vi "EthernetIP_CompactLogix_Servo.vi"() -> ()   [LabVIEW 2013]
uses:
  <vilib>/ethernetip/ethernetip.lvlib
  <vilib>/ethernetip/ethernetip.llb/EthernetIP Tag Write BOOL.vi
  <vilib>/ethernetip/ethernetip.llb/EthernetIP Tag Write REAL.vi
  <vilib>/ethernetip/ethernetip.llb/EthernetIP Tag Write DINT.vi
  <vilib>/ethernetip/ethernetip.llb/EthernetIP Tag Read BOOL.vi
panel:
  in  "Number of Elements 2":u32=1
  out "Servo1 Fault":bool
  in  "Number of Elements":u32=1
  out "Servo1 Fault":bool[](array[boolean])
  out "Servo1 Enabled":bool
  in  "VelocityLimit(172.20.2.53)":dbl=100.0
  in  "DecelerationLimit(172.20.2.53)":dbl=500.0
  in  "AccelerationLimit(172.20.2.53)":dbl=500.0
  in  "VelocityLimit(172.20.2.52)":dbl=100.0
  in  "DecelerationLimit(172.20.2.52)":dbl=500.0
  in  "AccelerationLimit(172.20.2.52)":dbl=500.0
  in  "Reference Source(172.20.2.53)":u16(ring)=3 items=["current", "velocity", "incremental position", "absolute position", "incremental registration", "absolute registration"]
  in  "Reference Source(172.20.2.52)":u16(ring)=3 items=["current", "velocity", "incremental position", "absolute position", "incremental registration", "absolute registration"]
  out "난수 결과값":dbl
  in  "CommandPosition":dbl(slide) scale=0.0..7.5
  in  "Time Delay":i32(knob)=50 scale=0.0..1000.0
  in  "StartMotion SW":bool
  in  "정지 버튼":bool
  in  "Error In":errorcluster caption="에러 입력"
  out "Error Out":errorcluster caption="에러 출력"
  in  "타임아웃":i32(knob)=1000 scale=0.0..1000.0
  in  "Servo1 On SW":bool
  # "Servo1(172.20.2.53)"
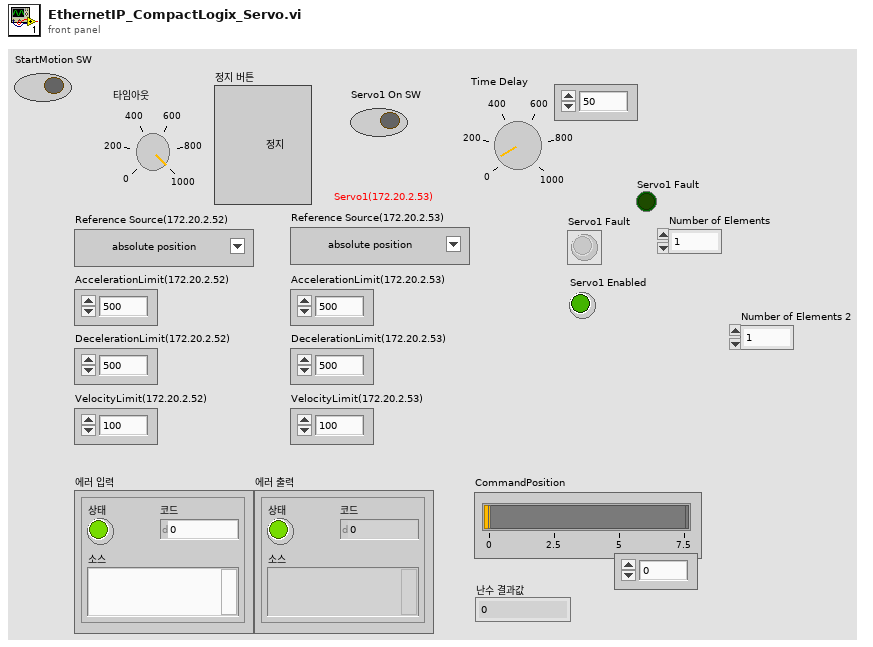
[diagram p1: front panel]
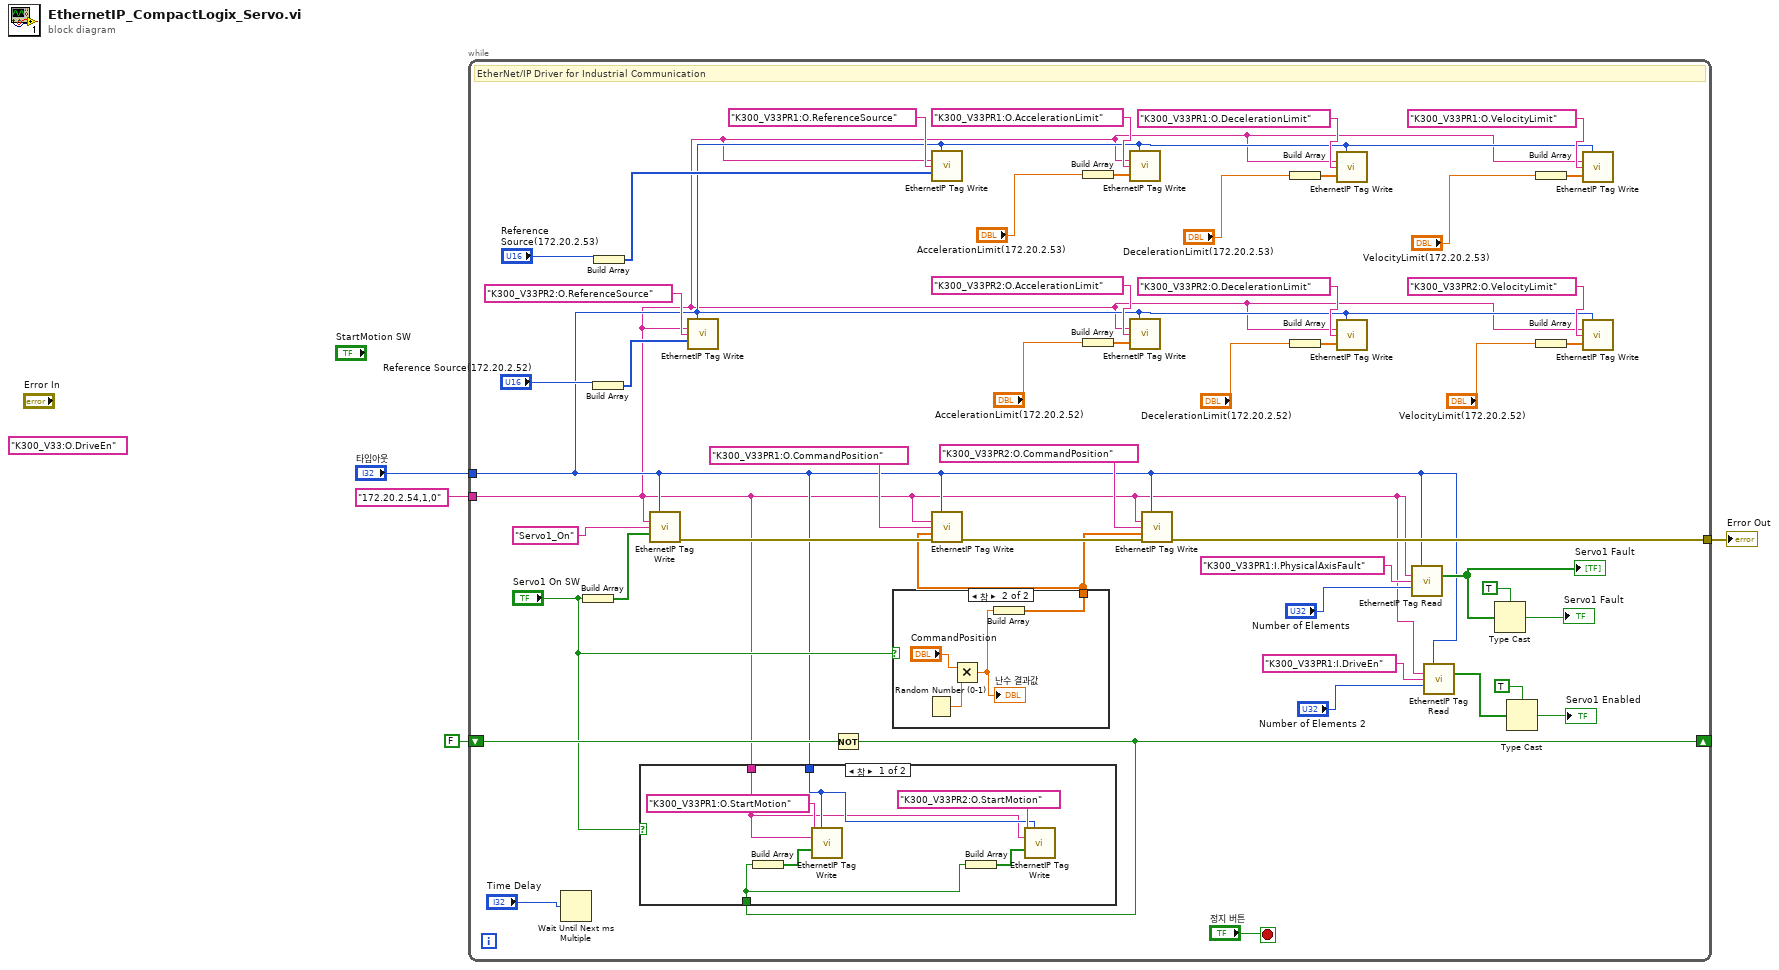
[diagram p0: block diagram]
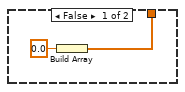
[diagram p2: hidden frame]
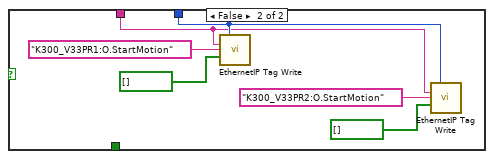
[diagram p3: hidden frame]
diagram:
  (unwired) "K300_V33:O.DriveEn" ("Tag Name")
  n1 = while {
    tunnel: [w48] -> w4
    shift-right: [w42] -> _
    shift-left: FALSE -> [w46]
    tunnel: "172.20.2.54,1,0" ("Network Path") -> [w6]
    tunnel: "타임아웃" -> [w7]
    stop <- "정지 버튼" stop-if-true
    # "EtherNet/IP Driver for Industrial Communication"
    n2 = Wait Until Next ms Multiple(millisecond multiple="Time Delay") -> ()  [unwired: 1 out]
    n3 = Build Array("Servo1 On SW") -> (w53:bool[])
    n4 = Build Array("Reference Source(172.20.2.52)") -> (w39:u16[])
    n5 = Build Array("Reference Source(172.20.2.53)") -> (w20:u16[])
    n6 = call-poly <vilib>:"EthernetIP Tag Write.vi"("Timeout (ms)"=w7, "Network Path"=w6, "Tag Name"="Servo1_On", "Data"=w53) -> ("error out"=w50:errorcluster)  [unwired: 10 in, 1 out]
    n7 = call-poly <vilib>:"EthernetIP Tag Write.vi"("Timeout (ms)"=w7, "Network Path"=w6, "Tag Name"="K300_V33PR2:O.ReferenceSource", "Data"=w39) -> ()  [unwired: 10 in, 2 out]
    n8 = Not(x=w46) -> (.not. x?=w42:bool)
    n9 = case shown="참" "Servo1 On SW" {
      tunnel: w42 -> [w60 _]
      tunnel: w7 -> [w62 w68]
      tunnel: w6 -> [w61 w67]
      frame True {
        n10 = Build Array(w60) -> (w65:bool[])
        n11 = call-poly <vilib>:"EthernetIP Tag Write.vi"("Timeout (ms)"=w62, "Network Path"=w61, "Tag Name"="K300_V33PR1:O.StartMotion", "Data"=w65) -> ()  [unwired: 10 in, 2 out]
        n12 = Build Array(w60) -> (w64:bool[])
        n13 = call-poly <vilib>:"EthernetIP Tag Write.vi"("Timeout (ms)"=w62, "Network Path"=w61, "Tag Name"="K300_V33PR2:O.StartMotion", "Data"=w64) -> ()  [unwired: 10 in, 2 out]
      }
      frame False {
        n14 = call-poly <vilib>:"EthernetIP Tag Write.vi"("Timeout (ms)"=w68, "Network Path"=w67, "Tag Name"="K300_V33PR1:O.StartMotion", "Data"=bool[] []) -> ()  [unwired: 10 in, 2 out]
        n15 = call-poly <vilib>:"EthernetIP Tag Write.vi"("Timeout (ms)"=w68, "Network Path"=w67, "Tag Name"="K300_V33PR2:O.StartMotion", "Data"=bool[] []) -> ()  [unwired: 10 in, 2 out]
      }
    }
    n16 = case shown="참" "Servo1 On SW" {
      tunnel: [w55 w56] -> w43
      frame False {
        n17 = Build Array(0.0 ("원소")) -> (w55:dbl[])
      }
      frame True {
        n18 = Random Number (0-1)() -> (number: 0 to 1=w59:dbl)
        n19 = Multiply(x="CommandPosition", y=w59) -> (x*y=w57:dbl)
        "난수 결과값" <- w57
        n20 = Build Array(w57) -> (w56:dbl[])
      }
    }
    n21 = call-poly <vilib>:"EthernetIP Tag Write.vi"("Timeout (ms)"=w7, "Network Path"=w6, "Tag Name"="K300_V33PR1:O.ReferenceSource", "Data"=w20) -> ()  [unwired: 10 in, 2 out]
    n22 = call-poly <vilib>:"EthernetIP Tag Write.vi"("Timeout (ms)"=w7, "Network Path"=w6, "Tag Name"="K300_V33PR1:O.CommandPosition", "Data"=w43, "error in"=w50) -> ("error out"=w49:errorcluster)  [unwired: 9 in, 1 out]
    n23 = Build Array("AccelerationLimit(172.20.2.53)") -> (w23:dbl[])
    n24 = Build Array("AccelerationLimit(172.20.2.52)") -> (w35:dbl[])
    n25 = call-poly <vilib>:"EthernetIP Tag Write.vi"("Timeout (ms)"=w7, "Network Path"=w6, "Tag Name"="K300_V33PR1:O.AccelerationLimit", "Data"=w23) -> ()  [unwired: 10 in, 2 out]
    n26 = call-poly <vilib>:"EthernetIP Tag Write.vi"("Timeout (ms)"=w7, "Network Path"=w6, "Tag Name"="K300_V33PR2:O.AccelerationLimit", "Data"=w35) -> ()  [unwired: 10 in, 2 out]
    n27 = call-poly <vilib>:"EthernetIP Tag Write.vi"("Timeout (ms)"=w7, "Network Path"=w6, "Tag Name"="K300_V33PR2:O.CommandPosition", "Data"=w43, "error in"=w49) -> ("error out"=w48:errorcluster)  [unwired: 9 in, 1 out]
    n28 = Build Array("DecelerationLimit(172.20.2.53)") -> (w24:dbl[])
    n29 = Build Array("DecelerationLimit(172.20.2.52)") -> (w32:dbl[])
    n30 = call-poly <vilib>:"EthernetIP Tag Write.vi"("Timeout (ms)"=w7, "Network Path"=w6, "Tag Name"="K300_V33PR1:O.DecelerationLimit", "Data"=w24) -> ()  [unwired: 10 in, 2 out]
    n31 = call-poly <vilib>:"EthernetIP Tag Write.vi"("Timeout (ms)"=w7, "Network Path"=w6, "Tag Name"="K300_V33PR2:O.DecelerationLimit", "Data"=w32) -> ()  [unwired: 10 in, 2 out]
    n32 = call-poly <vilib>:"EthernetIP Tag Read.vi"("Timeout (ms)"=w7, "Network Path"=w6, "Tag Name"="K300_V33PR1:I.PhysicalAxisFault", "Number of Elements"="Number of Elements") -> ("Data"=w12:bool[])  [unwired: 9 in, 2 out]
    "Servo1 Fault" <- w12
    n33 = call-poly <vilib>:"EthernetIP Tag Read.vi"("Timeout (ms)"=w7, "Network Path"=w6, "Tag Name"="K300_V33PR1:I.DriveEn", "Number of Elements"="Number of Elements 2") -> ("Data"=w11:bool[])  [unwired: 9 in, 2 out]
    n34 = Type Cast(type=TRUE, x=w12) -> (*(type *) &x=→"Servo1 Fault":bool)
    n35 = Type Cast(type=TRUE, x=w11) -> (*(type *) &x=→"Servo1 Enabled":bool)
    n36 = Build Array("VelocityLimit(172.20.2.53)") -> (w27:dbl[])
    n37 = Build Array("VelocityLimit(172.20.2.52)") -> (w29:dbl[])
    n38 = call-poly <vilib>:"EthernetIP Tag Write.vi"("Timeout (ms)"=w7, "Network Path"=w6, "Tag Name"="K300_V33PR1:O.VelocityLimit", "Data"=w27) -> ()  [unwired: 10 in, 2 out]
    n39 = call-poly <vilib>:"EthernetIP Tag Write.vi"("Timeout (ms)"=w7, "Network Path"=w6, "Tag Name"="K300_V33PR2:O.VelocityLimit", "Data"=w29) -> ()  [unwired: 10 in, 2 out]
  }
  "Error Out" <- w4
